vi "5.10 Low Pass Line Def.vi"(1 "Gains and Parameters":T1={"Control Gain"=0.0, "Line Setpoint in Pixels"=0.0, "Low Pass Gain"=0.0, "Image Low Pass Gain"=0.0, "Line Fullness Setpoint"=0.0, "Line Fullness Std"=0.1, "Max Filter Mod"=-10.0, "Fullness dev"=0.0}, 2 "Line Def In":T2) -> (0 "Low Pass Line Def Out":T2)   [LabVIEW 2010]
uses:
  6-OCU Neurons/6.10 Occipital Neurons/6.10.1 LineDef.ctl
  5.10 Algorithm Parameters and Controls.ctl
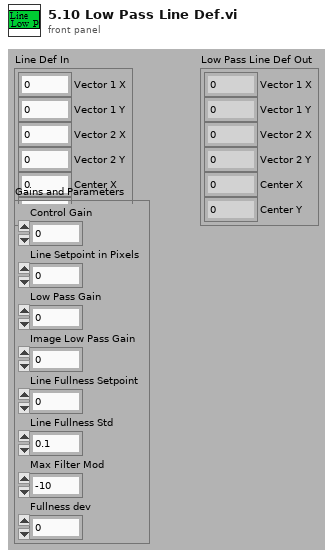
[diagram p1: front panel]
types:
  T1 = typedef "5.10 Algorithm Parameters and Controls.ctl" = cluster{"Control Gain":dbl, "Line Setpoint in Pixels":dbl, "Low Pass Gain":dbl, "Image Low Pass Gain":dbl, "Line Fullness Setpoint":dbl, "Line Fullness Std":dbl, "Max Filter Mod":dbl, "Fullness dev":dbl}
  T2 = typedef "6.10.1 LineDef.ctl" = cluster{"Vector 1 X":dbl, "Vector 1 Y":dbl, "Vector 2 X":dbl, "Vector 2 Y":dbl, "Center X":dbl, "Center Y":dbl}
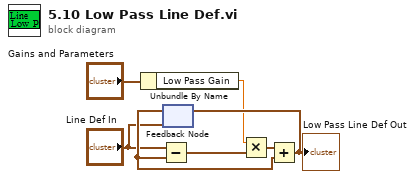
[diagram p0: block diagram]
diagram:
  n1 = Unbundle By Name("Gains and Parameters") -> ("Low Pass Gain"=w4:dbl)
  n2 = feedback #1("Line Def In") -> (w6:T2)
  n3 = Subtract(x="Line Def In", y=w6) -> (x-y=w1:T2)
  n4 = Multiply(x=w4, y=w1) -> (x*y=w2:T2)
  n5 = Add(x=w2, y=w6) -> (x+y=w7:T2)
  "Low Pass Line Def Out" <- w7
  n6 = feedback-in #1(w7) -> ()
